vi "Write Config File Path.vi"(8 "error in (no error)":errorcluster, 10 "config file path":path, 11 "[C] User Management in":refnum<class "[C] User Management.lvclass">) -> (0 "error out":errorcluster, 3 "[C] User Management out":refnum<class "[C] User Management.lvclass">)   [LabVIEW 2020, in "[C] User Management.lvlib" / "[C] User Management.lvclass"]
uses:
  [C] User Management.lvclass
  [C] User Management.lvclass/[C] User Management.ctl
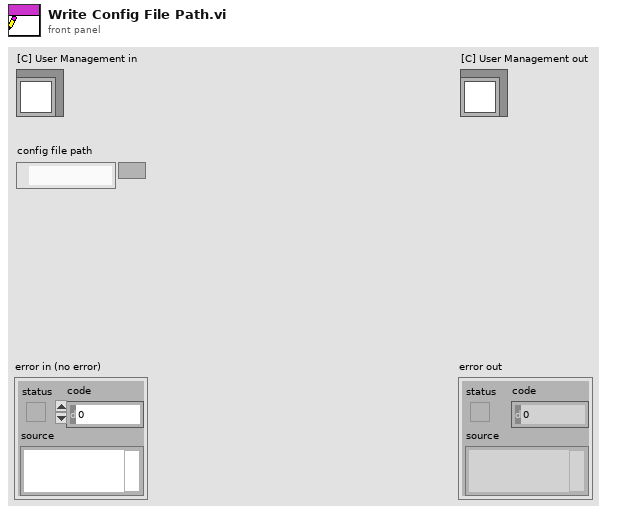
[diagram p1: front panel]
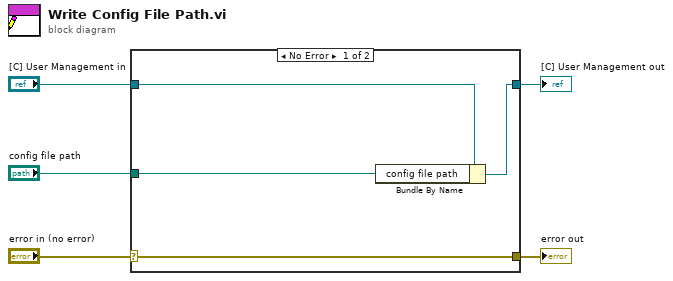
[diagram p0: block diagram]
diagram:
  n1 = case shown="No Error" "error in (no error)" {
    selector: "error in (no error)" -> [w9 w10]
    tunnel: [w9 w10] -> w4
    tunnel: [w7 w11] -> w2
    tunnel: "[C] User Management in" -> [w8 w11]
    tunnel: "config file path" -> [w6 _]
    frame No Error {
      n2 = Bundle By Name(cluster=w8, "config file path"=w6) -> (w7:refnum<class "[C] User Management.lvclass">)
    }
    frame Error {
    }
  }
  "error out" <- w4
  "[C] User Management out" <- w2
